vi "Dawson's Integral.vi"(3 "x":dbl format="%.2f") -> (1 "daw(x)":dbl format="%.2f")   [LabVIEW 2017, in "NI_Gmath.lvlib"]
doc: "Computes the Dawson integral."
uses:
  NI_Gmath.lvlib
  lvanlys.dll
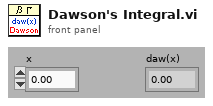
[diagram p1: front panel]
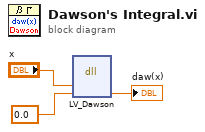
[diagram p0: block diagram]
diagram:
  n1 = dll-call lib="C:/Program Files/National Instruments/LabVIEW 2017/resource/lvanlys.*" fn="LV_Dawson"("x"="x", "dawson(x)"=0.0 ("Erf")) -> ("dawson(x)"=→"daw(x)":dbl)  [unwired: 5 in, 2 out]
